vi "And3 17.vi"(1 "C":bool, 2 "B":bool, 3 "A":bool) -> (0 "out":bool)   [LabVIEW 2018]
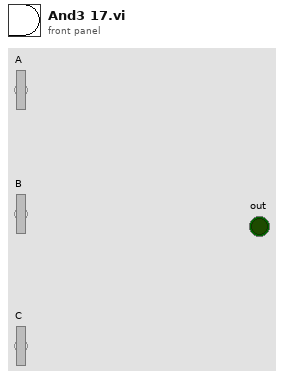
[diagram p1: front panel]
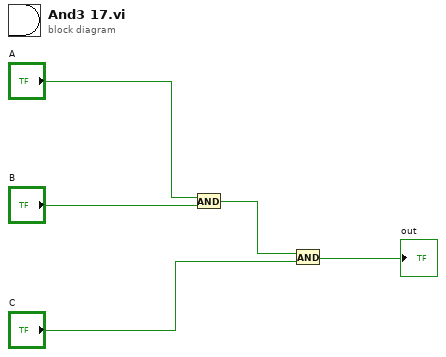
[diagram p0: block diagram]
diagram:
  n1 = And(x="A", y="B") -> (x .and. y?=w3:bool)
  n2 = And(x=w3, y="C") -> (x .and. y?=→"out":bool)
